vi "FindControlByName.vi"(8 "error in (no error)":errorcluster, 10 "Control_name":string, 11 "VI Refnum":refnum<vi>) -> (0 "error out":errorcluster, 3 "reference out":refnum<vi>)   [LabVIEW 2012]
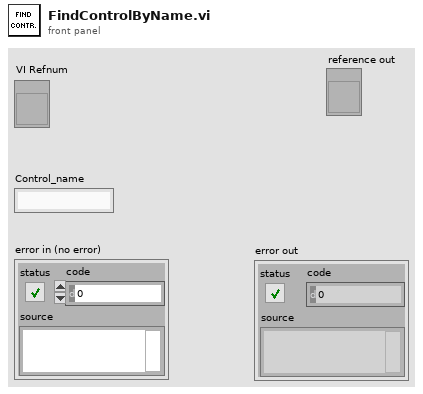
[diagram p1: front panel]
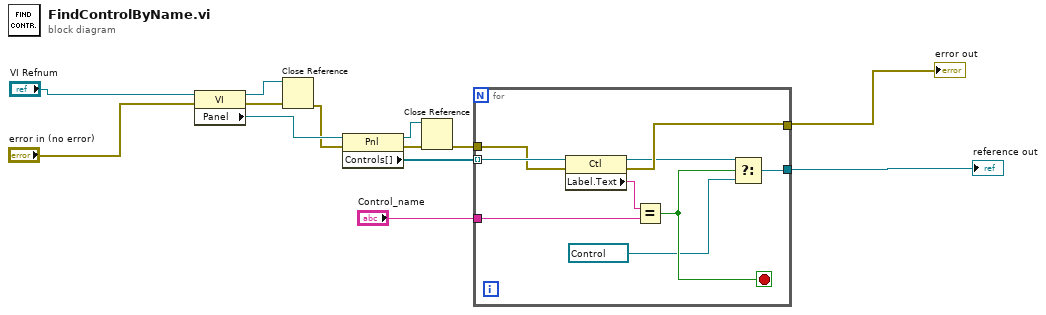
[diagram p0: block diagram]
diagram:
  n1 = property class="VI"(reference="VI Refnum", error in="error in (no error)") -> (reference out=w9:refnum<vi>, error out=w10:errorcluster, "Panel"=w11:refnum<vi>)
  n2 = Close Reference(reference=w9, error in (no error)=w10) -> (error out=w8:errorcluster)
  n3 = property class="Pnl"(reference=w11, error in=w8) -> (reference out=w6:refnum<vi>, error out=w7:errorcluster, "Controls[]"=w4:refnum<vi>[])
  n4 = Close Reference(reference=w6, error in (no error)=w7) -> (error out=w5:errorcluster)
  n5 = for {
    tunnel: w5 -> [w21]
    tunnel: w4 -> [w22] mode=indexing
    tunnel: "Control_name" -> [w19]
    tunnel: [w18] -> w2
    tunnel: [w15] -> w1
    stop <- w16 stop-if-true
    n6 = property class="Ctl"(reference=w22, error in=w21) -> (reference out=w17:refnum<vi>, error out=w18:errorcluster, "Label.Text"=w20:string)
    n7 = Equal?(x=w20, y=w19) -> (x = y?=w16:bool)
    n8 = Select(t=w17, s=w16, f=refnum<vi> refnum ("reference out")) -> (s? t:f=w15:refnum<vi>)
  }
  "error out" <- w2
  "reference out" <- w1
